vi "TDK_Set_Volt_Curr.vi"(7 "Power ON/OFF":bool=TRUE, 8 "error":errorcluster, 9 "Current Limit":dbl format="%.4f", 10 "Voltage Limit":dbl format="%.4f", 11 "VISA":refnum<visa-resource-name>="COM1") -> (0 "error out":errorcluster, 3 "VISA out":refnum<visa-resource-name>)   [LabVIEW 2016]
panel:
  in  "GEN Addr":i16=6
  # "Right-Click to\nexplain error"
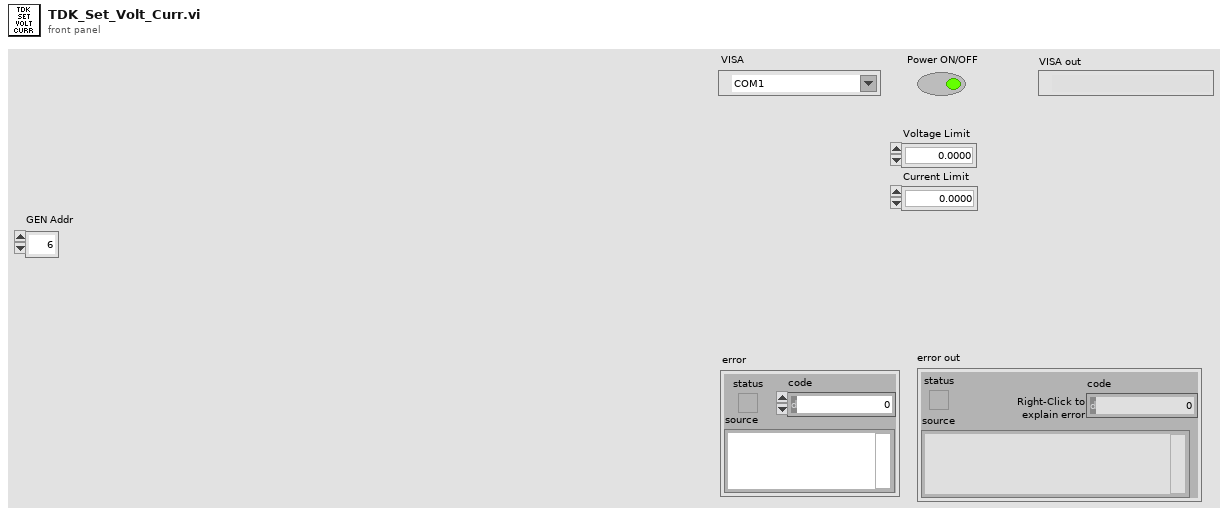
[diagram p1: front panel]
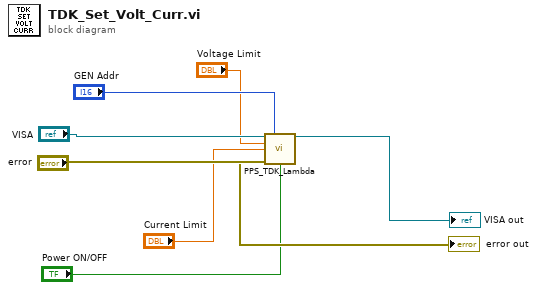
[diagram p0: block diagram]
diagram:
  n1 = call "PPS_TDK_Lambda.vi"("VISA"="VISA", "GEN Addr"="GEN Addr", "Voltage Limit"="Voltage Limit", "Current Limit"="Current Limit", "error"="error", "Output On (T)"="Power ON/OFF") -> ("VISA out"=→"VISA out":refnum<visa-resource-name>, "error out"=→"error out":errorcluster)  [unwired: 6 in, 2 out]
